vi "add ROI element.vi"(6 "new ROI in":T2[](array[typedef]) {"Contours"."Type" items=["No Selection", "Point", "Line", "Rectangle", "Oval", "Polygon", "Freehand Region", "Annulus", "Unused2", "Unused3", "Broken Line", "Freehand Line", "Rotated Rectangle"]}, 8 "错误输入（无错误）":errorcluster, 9 "image ROI in":T2[](array[typedef]) {"Contours"."Type" items=["No Selection", "Point", "Line", "Rectangle", "Oval", "Polygon", "Freehand Region", "Annulus", "Unused2", "Unused3", "Broken Line", "Freehand Line", "Rotated Rectangle"]}, 10 "new mask in":T1[](array[typedef]), 11 "image mask  in":T1[](array[typedef])) -> (0 "错误输出":errorcluster, 1 "image ROI out":T2[](array[typedef]) {"Contours"."Type" items=["No Selection", "Point", "Line", "Rectangle", "Oval", "Polygon", "Freehand Region", "Annulus", "Unused2", "Unused3", "Broken Line", "Freehand Line", "Rotated Rectangle"]}, 2 "ROI Descriptor out":T2 {"Contours"."Type" items=["No Selection", "Point", "Line", "Rectangle", "Oval", "Polygon", "Freehand Region", "Annulus", "Unused2", "Unused3", "Broken Line", "Freehand Line", "Rotated Rectangle"]}, 3 "image mask out":T1[](array[typedef]))   [LabVIEW 2013]
uses:
  <vilib>/vision/Image Controls.llb/IMAQ Image.ctl
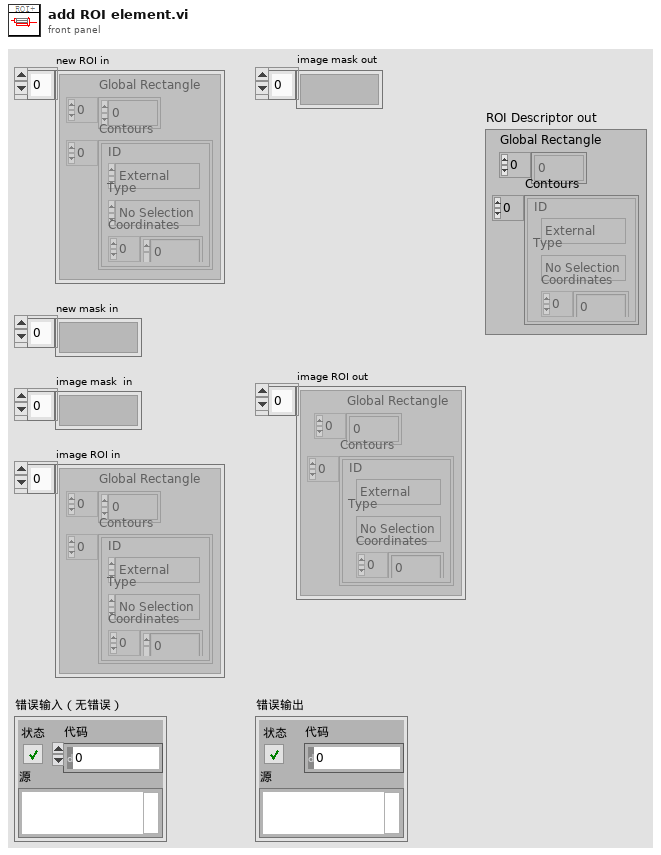
[diagram p1: front panel]
types:
  T1 = typedef "IMAQ Image.ctl" = refnum<image>
  T2 = typedef "ROI Descriptor" = cluster{"Global Rectangle":i32[], "Contours":cluster{"ID":enum32{"External", "Internal"}, "Type":u32, "Coordinates":i32[]}[]}
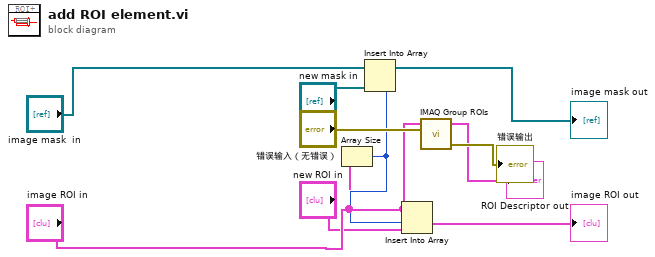
[diagram p0: block diagram]
diagram:
  n1 = Array Size(array="image ROI in") -> (size(s)=w6:i32)
  n2 = Insert Into Array(array="image mask  in", index=w6, new element="new mask in") -> (→"image mask out":T1[])
  n3 = Insert Into Array(array="image ROI in", index=w6, new element="new ROI in") -> (w7:T2[])
  "image ROI out" <- w7
  n4 = call "IMAQ Group ROIs"("error in (no error)"="错误输入（无错误）", "ROI Descriptors"=w7) -> ("error out"=→"错误输出":errorcluster, "ROI Descriptor out"=→"ROI Descriptor out":T2)  [unwired: 2 in]
